vi "sub vi - Strain Gauge Single.vi"(8 "rate":dbl=500.0 format="%0.2f", 9 "# of Samples":i32=500, 10 "timeout":dbl=70.0 format="%0.2f", 11 "Strain Gauge":tag="Dev1/ai27") -> (2 "mean":dbl format="%0.2f")   [LabVIEW 2010]
uses:
  <vilib>/DAQmx/read.llb/DAQmx Read (Analog 1D DBL 1Chan NSamp).vi
  <vilib>/DAQmx/create/channels.llb/DAQmx Create Channel (AI-Voltage-Basic).vi
  <vilib>/DAQmx/configure/timing.llb/DAQmx Timing (Sample Clock).vi
  <vilib>/daqmx/miscellaneous.llb/DAQmx Fill In Error Info.vi
  <vilib>/Analysis/NI_AALBase.lvlib
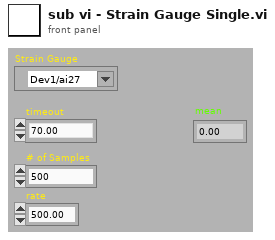
[diagram p1: front panel]
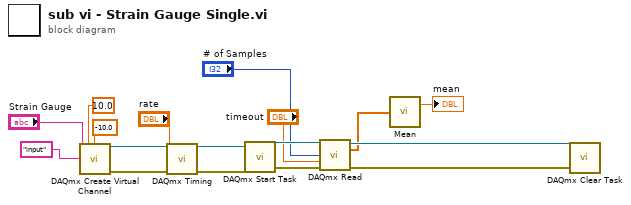
[diagram p0: block diagram]
diagram:
  n1 = call-poly <vilib>:"DAQmx Create Virtual Channel.vi"("maximum value"=10.0, "minimum value"=-10.0, "physical channels"="Strain Gauge", "name to assign"="input") -> ("task out"=w9:refnum<k21>, "error out"=w3:errorcluster)  [unwired: 5 in, 5 out]
  n2 = call-poly <vilib>:"DAQmx Timing.vi"("task/channels in"=w9, "rate"="rate", "error in"=w3) -> ("task out"=w4:refnum<k21>, "error out"=w2:errorcluster)  [unwired: 4 in, 7 out]
  n3 = call <vilib>:"DAQmx Start Task.vi"("task/channels in"=w4, "error in"=w2) -> ("task out"=w16:refnum<k21>, "error out"=w15:errorcluster)  [unwired: 12 out]
  n4 = call-poly <vilib>:"DAQmx Read.vi"("task/channels in"=w16, "number of samples per channel"="# of Samples", "timeout"="timeout", "error in"=w15) -> ("task out"=w12:refnum<k21>, "data"=w6:dbl[], "error out"=w11:errorcluster)  [unwired: 9 out]
  n5 = call <vilib>:"Mean.vi"("X"=w6) -> ("mean"=→"mean":dbl)  [unwired: 1 out]
  n6 = call <vilib>:"DAQmx Clear Task.vi"("task in"=w12, "error in"=w11) -> ()  [unwired: 14 out]
